vi "(SubVI) each theme index.vi"(1 "Theme compare":string[](array[string])) -> (0 "theme index":i32[][](array[numeric]))   [LabVIEW 2022 SP3]
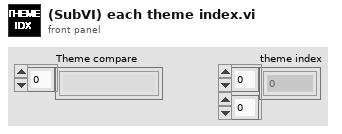
[diagram p1: front panel]
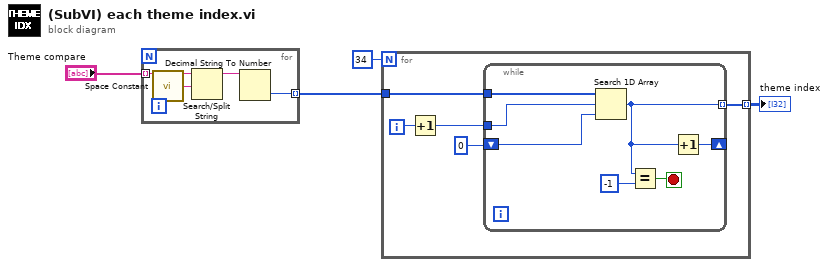
[diagram p0: block diagram]
diagram:
  n1 = for {
    tunnel: [w6] -> w4 mode=indexing
    tunnel: "Theme compare" -> [w5] mode=indexing
    n2 = call <vilib>:"Space Constant.vi"() -> ("String"=w8:string)
    n3 = Search/Split String(string=w5, search string/char (-)=w8) -> (substring before match=w7:string)  [unwired: 1 in, 2 out]
    n4 = Decimal String To Number(string=w7) -> (number=w6:i32)  [unwired: 2 in, 1 out]
  }
  n5 = for {
    N: 34 -> [_]
    tunnel: w4 -> [w13]
    tunnel: [w9] -> w1 mode=indexing
    i -> [w12]
    n6 = Increment(x=w12) -> (x+1=w11:i32)
    n7 = while {
      tunnel: w13 -> [w20]
      tunnel: w11 -> [w19]
      shift-right: [w16] -> _
      shift-left: 0 -> [w18]
      tunnel: [w15] -> w9 mode=indexing
      stop <- w14 stop-if-true
      n8 = Search 1D Array(1D array=w20, element=w19, start index (0)=w18) -> (index of element=w15:i32)
      n9 = Equal?(x=w15, y=-1) -> (x = y?=w14:bool)
      n10 = Increment(x=w15) -> (x+1=w16:i32)
    }
  }
  "theme index" <- w1
